vi "PulseGenerator.vi"(9 "TL":dbl, 11 "TH":dbl) -> (2 "Waveform Chart":dbl[](graph))   [LabVIEW 2022 SP3]
uses:
  <vilib>/Analysis/NI_AALPro.lvlib
panel:
  in  "amplitude":dbl=1.0 format="%0.2f"
  in  "signal type":T1(ring)
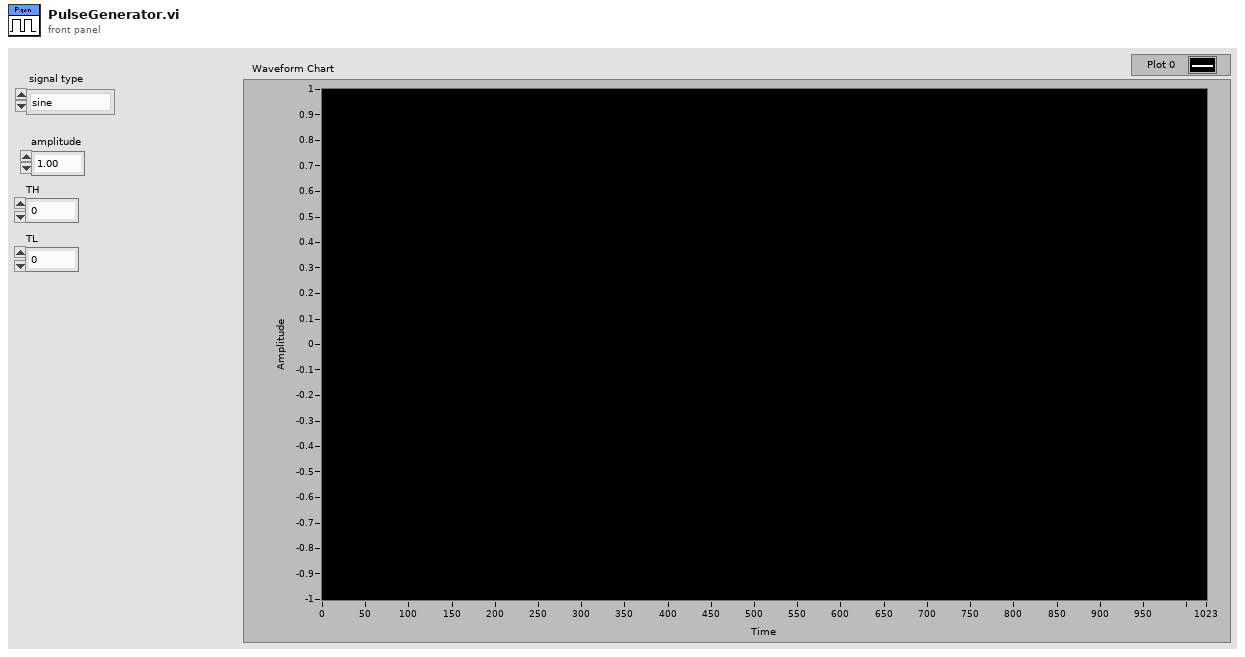
[diagram p1: front panel]
types:
  T1 = enum16{"sine", "cosine", "triangle", "square", "sawtooth", "increasing ramp", "decreasing ramp"}
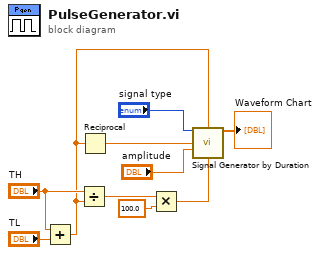
[diagram p0: block diagram]
diagram:
  n1 = Add(x="TH", y="TL") -> (x+y=w1:dbl)
  n2 = Divide(x="TH", y=w1) -> (x/y=w5:dbl)
  n3 = Reciprocal(x=w1) -> (1/x=w7:dbl)
  n4 = Multiply(x=w5, y=100.0) -> (x*y=w3:dbl)
  n5 = call <vilib>:"Signal Generator by Duration.vi"("signal type"="signal type", "duration"=w1, "frequency"=w7, "amplitude"="amplitude", "square wave duty cycle (%)"=w3) -> ("signal"=→"Waveform Chart":dbl[])  [unwired: 7 in, 3 out]
